vi "Load.vi"(8 "Error In":errorcluster, 10 "Key":string, 11 "Loader In":refnum<class "Loader.lvclass">) -> (0 "Error Out":errorcluster, 2 "Template":string, 3 "Loader Out":refnum<class "Loader.lvclass">)   [LabVIEW 2018, in "Toolkit.lvlib" / "Loaders.lvlib" / "Loader.lvclass"]
doc: "Gets a template as a string based on the Partial's key value in the root, or master, template.\n\n<B>Loader In/Out</B> - Represents an implementation capable of loading, or including, a partial Mustache template.\n\n<B>Key</B> - The key from the partial tag.\n\n<B>Template</B> - The partial Mustache template associated with the key. The origin of the template depends on the loader's implementation and the data type associated with the key."
uses:
  Loader.lvclass
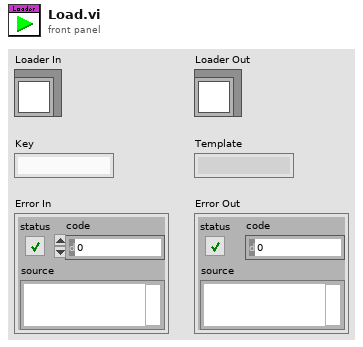
[diagram p1: front panel]
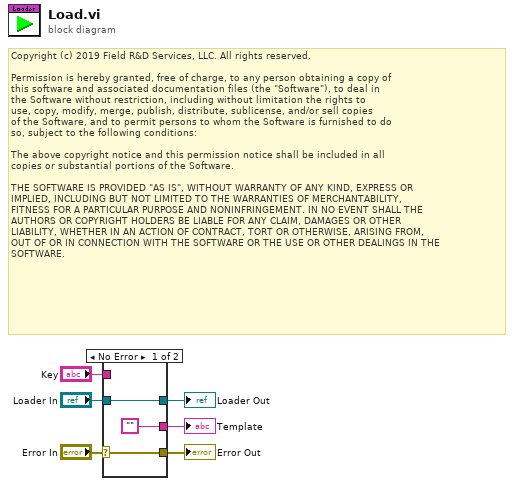
[diagram p0: block diagram]
diagram:
  # "Copyright (c) 2019 Field R&D Services, LLC. All rights reserved.\n\nPermission is hereby granted, free of charge, to any person obtaining a copy of\nthis software and associated documentation files (the \"Software\"), to deal in\nthe Software without restriction, including without limitation the rights to\nuse, copy, modify, merge, publish, distribute, sublicense, and/or sell copies\nof the Software, and to permit persons to whom the Software is furnished to do\nso, subject to the following conditions:\n\nThe above copyright notice and this permission notice shall be included in all\ncopies or substantial portions of the Software.\n\nTHE SOFTWARE IS PROVIDED \"AS IS\", WITHOUT WARRANTY OF ANY KIND, EXPRESS OR\nIMPLIED, INCLUDING BUT NOT LIMITED TO THE WARRANTIES OF MERCHANTABILITY,\nFITNESS FOR A PARTICULAR PURPOSE AND NONINFRINGEMENT. IN NO EVENT SHALL THE\nAUTHORS OR COPYRIGHT HOLDERS BE LIABLE FOR ANY CLAIM, DAMAGES OR OTHER\nLIABILITY, WHETHER IN AN ACTION OF CONTRACT, TORT OR OTHERWISE, ARISING FROM,\nOUT OF OR IN CONNECTION WITH THE SOFTWARE OR THE USE OR OTHER DEALINGS IN THE\nSOFTWARE."
  n1 = case shown="No Error" "Error In" {
    selector: "Error In" -> [w9 w10]
    tunnel: "Loader In" -> [w8 w11]
    tunnel: [w8 w11] -> w5
    tunnel: [w9 w10] -> w3
    tunnel: ["" _] -> w2
    tunnel: "Key" -> [_ _]
    frame No Error {
    }
    frame Error {
    }
  }
  "Loader Out" <- w5
  "Error Out" <- w3
  "Template" <- w2
